vi "Joint_Command_Mode.vi"(0 "Side":T1, 1 "node":string, 2 "Mode":u8(ring) items=["Position", "Velocity", "Effort"], 3 "error in":errorcluster) -> (6 "error out":errorcluster)   [LabVIEW 2010]
uses:
  <userlib>/ROSforLV_0.1/ROS/Code/SubVIs/BaxterSide.ctl
  <userlib>/ROSforLV_0.1/ROS/MessageBuilding/Primitives/subs/u8Scalar.vi
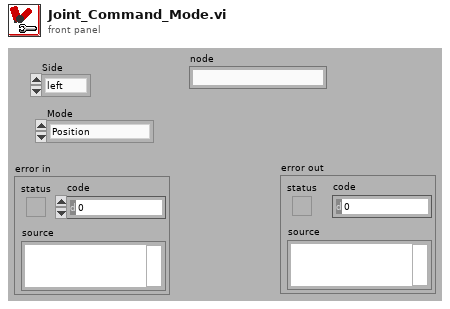
[diagram p1: front panel]
types:
  T1 = typedef "BaxterSide.ctl" = enum16{"left", "right"}
  T2 = typedef "_ROSControl.ctl" = cluster{"topic port":u16, "Node":string, "topic":string, "type":string, "node port":u32, "error ":errorcluster, "Direction":T3, "APIs":string[]}
  T3 = typedef "_ROSDirection.ctl" = enum16{"Node", "Publisher", "Subscriber", "Service Client"}
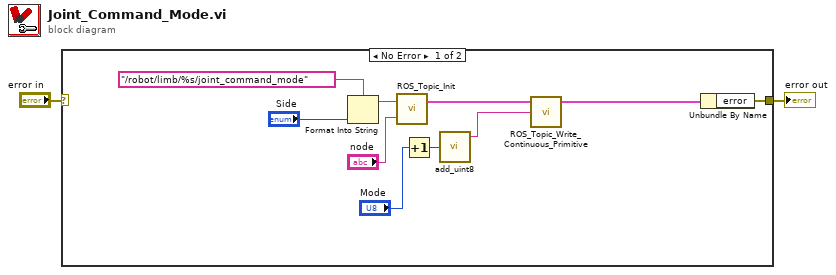
[diagram p0: block diagram]
diagram:
  n1 = case shown="No Error" "error in" {
    selector: "error in" -> [_ w13]
    tunnel: [w10 w13] -> w2
    frame No Error {
      n2 = Format Into String(format string="/robot/limb/%s/joint_command_mode" ("topic"), "Side") -> (resulting string=w7:string)  [unwired: 2 in, 1 out]
      n3 = call <userlib>:"ROS_Topic_Init.vi"("node"="node", "topic"=w7) -> ("ROS out"=w12:T2)  [unwired: 1 in]
      n4 = Increment(x="Mode") -> (x+1=w5:u8)
      n5 = call-poly <userlib>:"add_uint8.vi"("Numeric"=w5) -> ("msg out"=w4:string)  [unwired: 4 in]
      n6 = call <userlib>:"ROS_Topic_Write_Continuous_Primitive.vi"("Msg in"=w4, "ROS in"=w12) -> ("ROS out"=w11:T2)  [unwired: 3 in]
      n7 = Unbundle By Name(w11) -> ("error"=w10:errorcluster)
    }
    frame Error {
    }
  }
  "error out" <- w2
